vi "saveTargetsFile.vi"(5 "BL Targets":T1[](array[typedef])=[{"Code"="B2", "TI Profile (FS)"=[[15.0, 25.5], [20.0, 24.3], [25.0, 23.5], [30.0, 22.9], [35.0, 22.3], [45.0, 21.5], [55.0, 20.9], [65.0, 20.4], [80.0, 19.7], [100.0, 19.0], [125.0, 18.2], [150.0, 17.6], [200.0, 16.5], [235.0, 15.8], [300.0, 14.7], [360.0, 13.9]], "n"=0.23999999999999996}, {"Code"="C2", "TI Profile (FS)"=[[15.0, 16.0], [20.0, 15.6], [25.0, 15.2], [30.0, 14.9], [35.0, 14.7], [45.0, 14.2], [55.0, 13.9], [65.0, 13.5], [80.0, 13.0], [100.0, 12.5], [125.0, 11.9], [150.0, 11.4], [200.0, 10.5], [235.0, 10.0], [300.0, 9.2], [360.0, 8.6]], "n"=0.14}] {"n" min=0.02 max=0.5 step=0.01 format="%.2f"}, 7 "Path":path, 10 "Scale":dbl=300.0 caption="Scale 1:" min=1.0 max=10000.0 step=50.0) -> ()   [LabVIEW 2016]
uses:
  BLTarget.ctl
  Error bar Type.ctl
panel:
  out "String":string
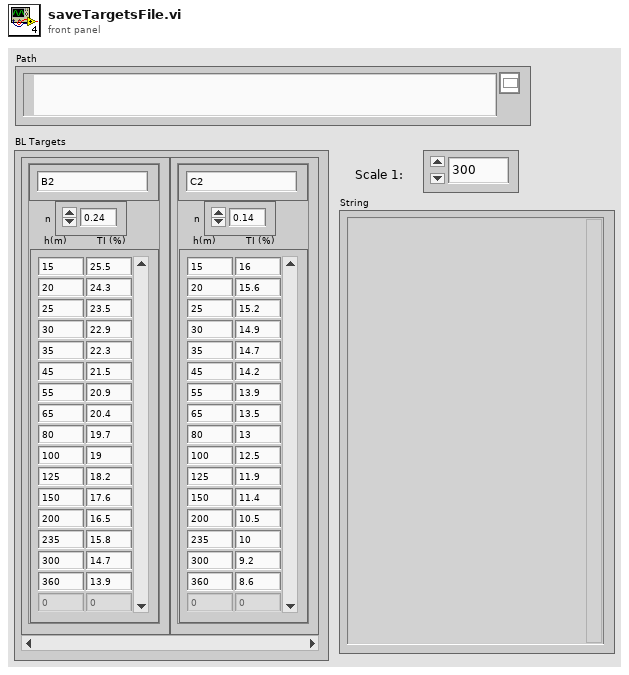
[diagram p1: front panel]
types:
  T1 = typedef "BLTarget.ctl" = cluster{"Code":string, "TI Profile (FS)":dbl[][], "n":dbl}
  T2 = typedef "Error bar Type.ctl" = enum16{"Standard Error", "Separate upper and lower"}
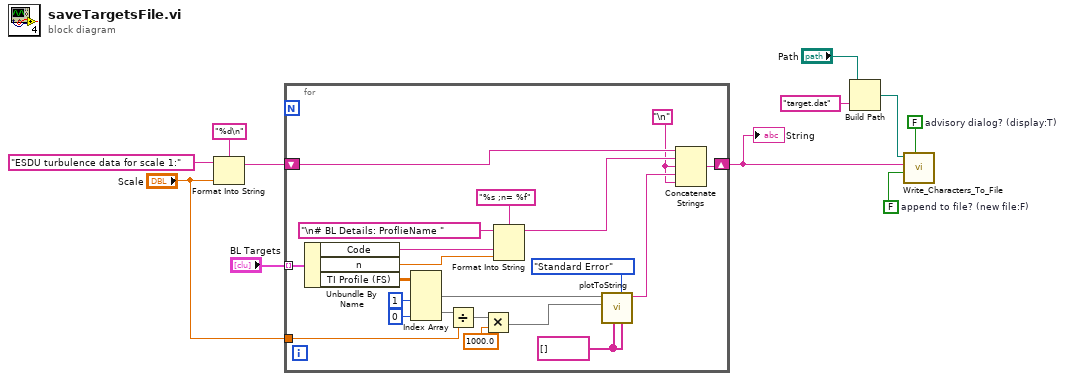
[diagram p0: block diagram]
diagram:
  w6 = FALSE  # advisory dialog? (display:T)
  w5 = FALSE  # append to file? (new file:F)
  n1 = Format Into String(format string="%d\n", initial string="ESDU turbulence data for scale 1:", "Scale") -> (resulting string=w8:string)  [unwired: 1 in, 1 out]
  n2 = for {
    tunnel: "BL Targets" -> [w32] mode=indexing
    shift-right: [w25] -> w2
    shift-left: w8 -> [w26]
    tunnel: "Scale" -> [w18]
    w13 = string[] [] ("Error Bar values")
    w14 = "\n"
    n3 = Unbundle By Name(w32) -> ("Code"=w31:string, "n"=w30:dbl, "TI Profile (FS)"=w19:dbl[][])
    n4 = Index Array(array=w19, index (col) #1=1 ("disabled index (col)"), index (col) #2=0 ("index (col)")) -> (element #1=w15:dbl[], element #2=w21:dbl[])  [unwired: 2 in]
    n5 = Divide(x=w21, y=w18) -> (x/y=w22:dbl[])
    n6 = Multiply(x=w22, y=1000.0) -> (x*y=w16:dbl[])
    n7 = Format Into String(format string="%s ;n= %f", initial string="\n# BL Details: ProflieName ", w31, w30) -> (resulting string=w27:string)  [unwired: 1 in, 1 out]
    n8 = call "plotToString.vi"("Error Bar upper"=w13, "Error Bar Type"=Error_bar_Type."Standard Error", "Error Bar lower"=w13, "Column2"=w16, "Column1"=w15) -> ("plotString"=w17:string)  [unwired: 5 in, 1 out]
    n9 = Concatenate Strings(w26, w27, w14, w17, w14) -> (w25:string)
  }
  "String" <- w2
  n10 = Build Path(base path="Path", name or relative path="target.dat") -> (appended path=w3:path)
  n11 = call "Write_Characters_To_File.vi"("file path (dialog if empty)"=w3, "advisory dialog? (display:T)"=w6, "character string"=w2, "append to file? (new file:F)"=w5) -> ()  [unwired: 1 in, 4 out]
